vi "MS SQL_InRFID_STN50B.vi"(6 "RFID":string, 7 "OP50B_011_BIC":T1, 8 "error in (no error)":errorcluster, 11 "Ref in":T2={"MS SQL Connection"=refnum, "UDL File"=path "", "Time"="", "DCODE"="", "WIP+1"=0, "MC No?"=0, "POKAYOKE?"=FALSE, "Expected Result"="", "Result [Status]"="", "Clock"=0.0, "RFID"="", "WIP Queue"=refnum, "TS Parameter"={"ProfitCenterCode"="", "LineCode"="", "WorkOrderNumber"="", "Model"="", "Model_with_Prefix"="", "VendorCode"="", "SetParameterDateCode"="", "PokaYoke"=0, "Target"=1, "Live_DateCode"="", "CustomerPartNumber"="", "Hand"="", "Ent_Stamp"=timestamp(0 s since 1904-01-01), "STS_CD"=0.0}, "Data_Queue"=[], "RFID Serial No."=""} {"TS Parameter"."Target" min=1 max=100000; "TS Parameter"."PokaYoke" min=0 max=1}) -> (0 "error out":errorcluster, 1 "Message":picture, 3 "Ref Out":T2={"MS SQL Connection"=refnum, "UDL File"=path "", "Time"="", "DCODE"="", "WIP+1"=0, "MC No?"=0, "POKAYOKE?"=FALSE, "Expected Result"="", "Result [Status]"="", "Clock"=0.0, "RFID"="", "WIP Queue"=refnum, "TS Parameter"={"ProfitCenterCode"="", "LineCode"="", "WorkOrderNumber"="", "Model"="", "Model_with_Prefix"="", "VendorCode"="", "SetParameterDateCode"="", "PokaYoke"=0, "Target"=1, "Live_DateCode"="", "CustomerPartNumber"="", "Hand"="", "Ent_Stamp"=timestamp(0 s since 1904-01-01), "STS_CD"=0.0}, "Data_Queue"=[], "RFID Serial No."=""} {"TS Parameter"."Target" min=1 max=100000; "TS Parameter"."PokaYoke" min=0 max=1})   [LabVIEW 2020]
uses:
  Controls/TD SQL.ctl
  <vilib>/addons/database/Connection.llb/Conn ObjectReference.ctl
  Controls/WIP_State.ctl
  Controls/TS_Parameter.ctl
  Controls/OP50B_DataCluster.ctl
  <vilib>/addons/database/NI_Database_API.lvlib
panel:
  out "resulting string":string
  # "OP80"
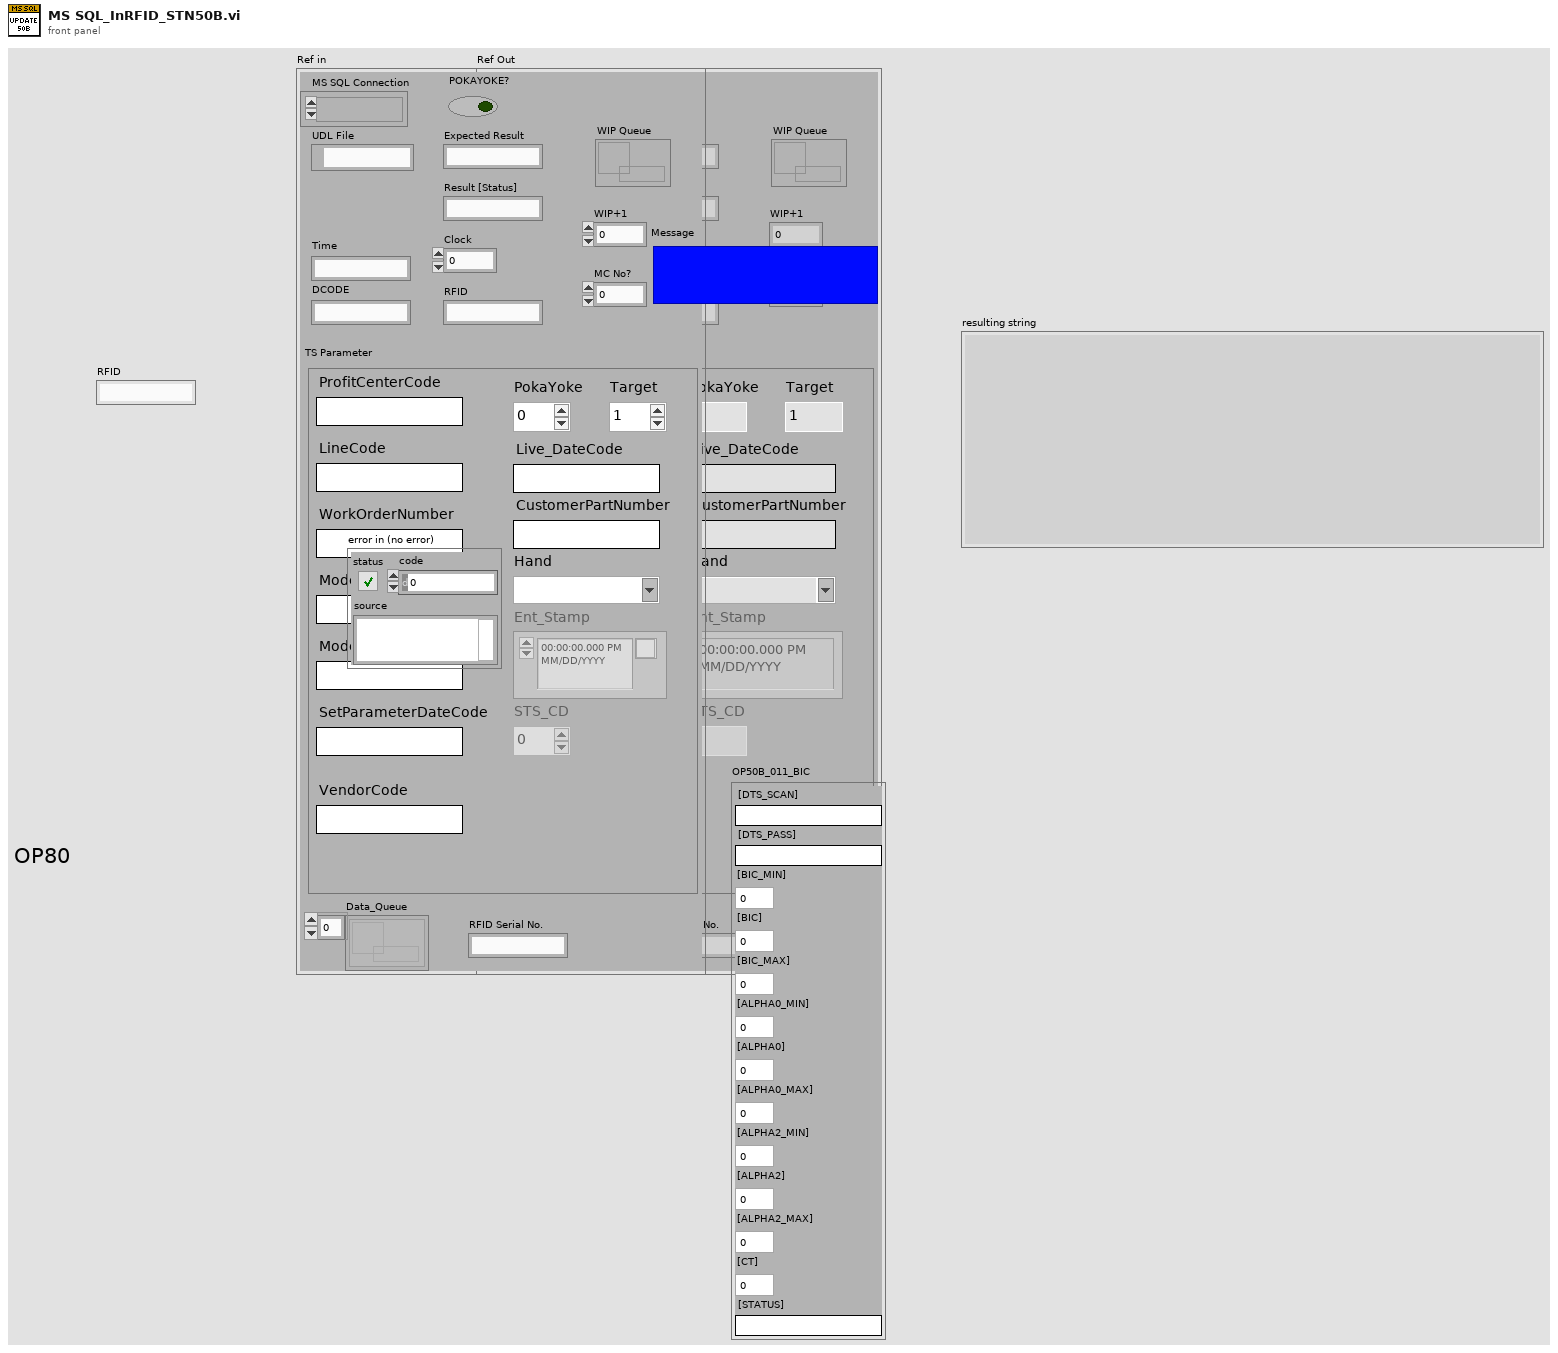
[diagram p1: front panel]
types:
  T1 = typedef "OP50B_DataCluster.ctl" = cluster{"[DTS_SCAN]":string, "[DTS_PASS]":string, "[BIC_MIN]":dbl, "[BIC]":dbl, "[BIC_MAX]":dbl, "[ALPHA0_MIN]":dbl, "[ALPHA0]":dbl, "[ALPHA0_MAX]":dbl, "[ALPHA2_MIN]":dbl, "[ALPHA2]":dbl, "[ALPHA2_MAX]":dbl, "[CT]":dbl, "[STATUS]":string}
  T2 = typedef "TD SQL.ctl" = cluster{"MS SQL Connection":T3, "UDL File":path, "Time":string, "DCODE":string, "WIP+1":i64, "MC No?":i32, "POKAYOKE?":bool, "Expected Result":string, "Result [Status]":string, "Clock":dbl, "RFID":string, "WIP Queue":refnum<queue>, "TS Parameter":T4, "Data_Queue":refnum<queue>[], "RFID Serial No.":string}
  T3 = typedef "NI_Database_API.lvlib/Conn ObjectReference.ctl" = refnum<k1>
  T4 = typedef "TS_Parameter.ctl" = cluster{"ProfitCenterCode":string, "LineCode":string, "WorkOrderNumber":string, "Model":string, "Model_with_Prefix":string, "VendorCode":string, "SetParameterDateCode":string, "PokaYoke":i32, "Target":i32, "Live_DateCode":string, "CustomerPartNumber":string, "Hand":string, "Ent_Stamp":timestamp, "STS_CD":dbl}
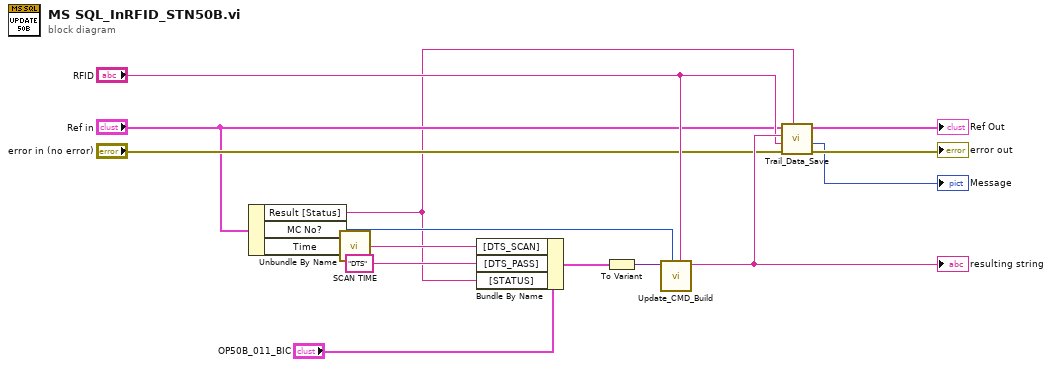
[diagram p0: block diagram]
diagram:
  n1 = Unbundle By Name("Ref in") -> ("Result [Status]"=w1:string, "MC No?"=w2:i32, "Time"=w3:string)
  n2 = call "SCAN TIME.vi"("Time in"=w3) -> ("Time out"=w12:string)
  n3 = Bundle By Name(cluster="OP50B_011_BIC", "[DTS_SCAN]"=w12, "[DTS_PASS]"="DTS", "[STATUS]"=w1) -> (w13:T1)
  n4 = To Variant(anything=w13) -> (Variant=w15:variant)
  n5 = call "Update_CMD_Build.vi"("RFID"="RFID", "Machine No"=w2, "Variant"=w15) -> ("Update Query"=w9:string)  [unwired: 5 in, 1 out]
  "resulting string" <- w9
  n6 = call "Trail_Data_Save.vi"("Status"=w1, "error in (no error)"="error in (no error)", "RFID"="RFID", "Query"=w9, "Ref in"="Ref in") -> ("error out"=→"error out":errorcluster, "Message"=→"Message":picture, "Ref Out"=→"Ref Out":T2)  [unwired: 1 in, 1 out]
